vi "Read Rubi spectra configuration.vi"(8 "error in (no error)":errorcluster, 11 "Ruby Spectra in":refnum<class "Ruby Spectra.lvclass">) -> (0 "error out":errorcluster, 2 "Rubi spectra configuration":T1={"Integration time"=0.5, "Fit parameters"={"Function"=enum."Gauss", "Window width"=0.0, "Initial guess"={"Amplitude"=1000.0, "Center"=694.3, "Width"=0.4}}, "Fit"=FALSE, "Auto-update params"=FALSE, "Save spectra"=FALSE, "Reference wavelengh"=694.123, "Background"=path ""} {"Reference wavelengh" format="%#_gnm"; "Fit parameters"."Initial guess"."Width" format="%#_gnm"; "Fit parameters"."Initial guess"."Center" format="%#_gnm"; "Fit parameters"."Window width" format="%#_6gnm"; "Integration time" format="%#_6ps"}, 3 "Ruby Spectra out":refnum<class "Ruby Spectra.lvclass">)   [LabVIEW 2018, in "Ruby Spectra.lvclass"]
uses:
  Ruby Spectra.lvclass
  C:/github/2018/LabActor/Template Module/Template Module.lvclass
  NHMFL_Core/Libraries/Instruments/Ocean Optics/Ocean Optics Driver/Ocean optics configuration.ctl
  NHMFL_Core/Libraries/Utilities/Fit/Multi-peak Parameters.ctl
  NHMFL_Core/Libraries/Utilities/Fit/Peak Parameters.ctl
  Template Module/Template Module.lvclass/Template Module.ctl
  Template Module/Read Configuration.vi
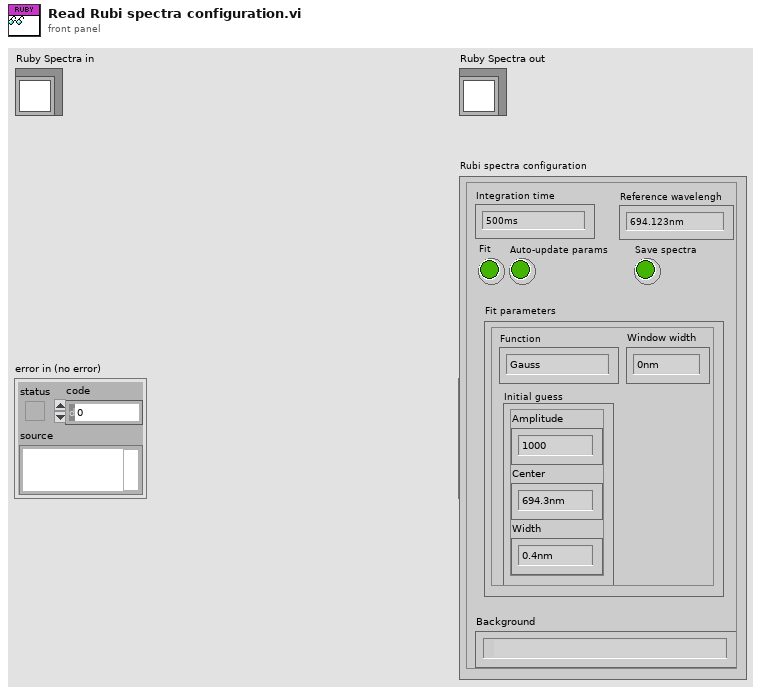
[diagram p1: front panel]
types:
  T1 = typedef "Ruby Spectra.lvclass/Ocean optics configuration.ctl" = cluster{"Integration time":dbl, "Fit parameters":T2, "Fit":bool, "Auto-update params":bool, "Save spectra":bool, "Reference wavelengh":dbl, "Background":path}
  T2 = typedef "Multi-peak Parameters.ctl" = cluster{"Function":enum16{"Gauss", "Lorentz"}, "Window width":dbl, "Initial guess":T3}
  T3 = typedef "Peak Parameters.ctl" = cluster{"Amplitude":dbl, "Center":dbl, "Width":dbl}
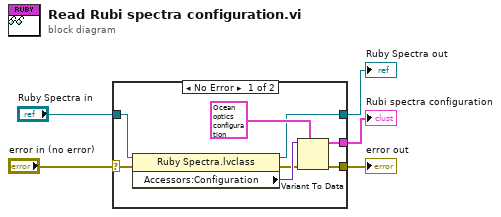
[diagram p0: block diagram]
diagram:
  n1 = case shown="No Error" "error in (no error)" {
    selector: "error in (no error)" -> [w13 w14]
    tunnel: [w7 w14] -> w4
    tunnel: [w10 w15] -> w2
    tunnel: "Ruby Spectra in" -> [w11 w15]
    tunnel: [w6 _] -> w1
    frame No Error {
      n2 = property class="Ruby Spectra.lvclass"(reference=w11, error in=w13) -> (reference out=w10:refnum<class "Ruby Spectra.lvclass">, error out=w8:errorcluster, "Accessors:Configuration"=w9:variant)
      n3 = Variant To Data(error in=w8, type=T1 {"Integration time"=0.5, "Fit parameters"={"Function"=enum."Gauss", "Window width"=0.0, "Initial guess"={"Amplitude"=1000.0, "Center"=694.3, "Width"=0.4}}, "Fit"=TRUE, "Auto-update params"=FALSE, "Save spectra"=FALSE, "Reference wavelengh"=694.123, "Background"=path ""} ("Rubi spectra configuration"), Variant=w9) -> (data=w6:T1, error out=w7:errorcluster)
    }
    frame Error {
    }
  }
  "error out" <- w4
  "Ruby Spectra out" <- w2
  "Rubi spectra configuration" <- w1
